vi "Adv_ReadQueueReference.vi"(11 "LightField Automation in":refnum<class "LightField Automation.lvclass">) -> (2 "Queue Reference":refnum<queue>, 3 "LightField Automation out":refnum<class "LightField Automation.lvclass">)   [LabVIEW 2015, in "LightField Automation.lvclass"]
uses:
  LightField Automation.lvclass
  LightField Automation.lvclass/LightField Automation.ctl
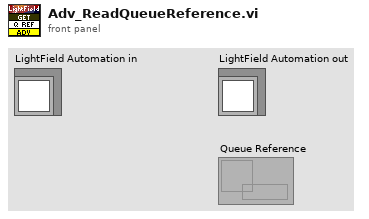
[diagram p1: front panel]
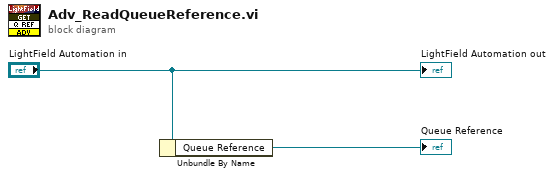
[diagram p0: block diagram]
diagram:
  n1 = Unbundle By Name("LightField Automation in") -> ("Queue Reference"=→"Queue Reference":refnum<queue>)
  "LightField Automation out" <- "LightField Automation in"
